vi "chipKIT UART2 Write.vi"() -> ()   [LabVIEW 2011, in "LabVIEW Interface for ChipKit.lvlib"]
doc: "Write serial data using the secondary UART on the chipKIT."
uses:
  vi.lib/LabVIEW Interface for ChipKit/LabVIEW Interface for ChipKit.lvlib
  vi.lib/LabVIEW Interface for ChipKit/Private/Type Defs/Chipkit Configuration.ctl
  vi.lib/LabVIEW Interface for ChipKit/Private/Type Defs/Board Type.ctl
panel:
  in  "Send":bool
  in  "Serial Data":string
  in  "Stop Button":bool
  in  "Buad Rate":u32=9600
  in  "ChipKit Configuration":T1={"COM Port"="COM3", "Board Type"=enum."ChipKit uC32"}
  # "UART2 Write Example\n\nThis example demonstrates how write serial data usring the secondary UART\non the chipKIT\n\nInstructions\n1. Select the COM Port associated with the ChipKit.\n2. Select the Board Type.\n3. Select the Baud Rate for thes secondary UART.\n4. Click the Run Arrow.\n5. Enter a value into the Serial Data string control.\n6. Click Send."
  # "chipKIT Settings"
  # "Channel Settings"
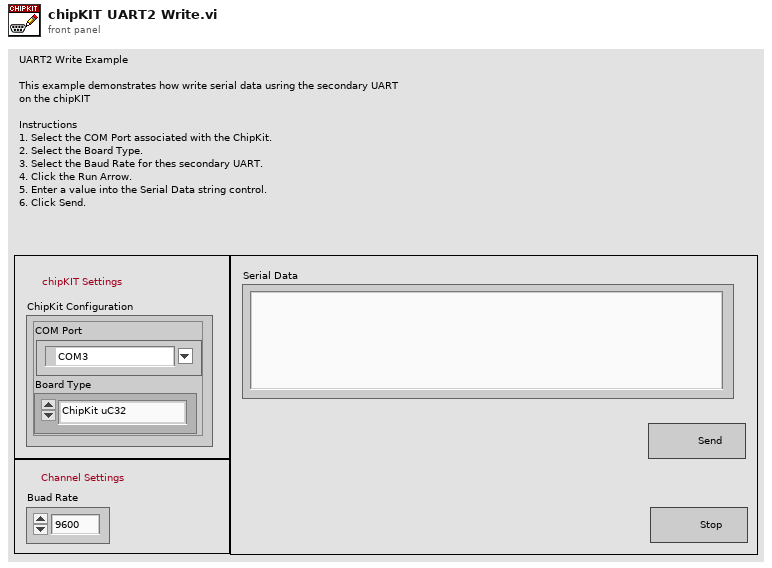
[diagram p1: front panel]
types:
  T1 = typedef "LabVIEW Interface for ChipKit.lvlib/Chipkit Configuration.ctl" = cluster{"COM Port":refnum<visa-resource-name>, "Board Type":T2}
  T2 = typedef "LabVIEW Interface for ChipKit.lvlib/Board Type.ctl" = enum16{"ChipKit uC32", "ChipKit Uno32", "ChipKit Max32"}
  T3 = typedef "LabVIEW Interface for ChipKit.lvlib/Chipkit Resource.ctl" = cluster{"COM Port":refnum<visa-resource-name>, "Board Type":T2, "Connection Type":T4, "Baud Rate (115200)":u32, "Bytes Per Packet (15)":u32, "DI Port Num Pins":i32, "DO Port Num Pins":i32}
  T4 = typedef "LabVIEW Interface for ChipKit.lvlib/Connection Type.ctl" = enum8{"USB / Serial", "XBEE", "BlueSmirf (Bluetooth)"}
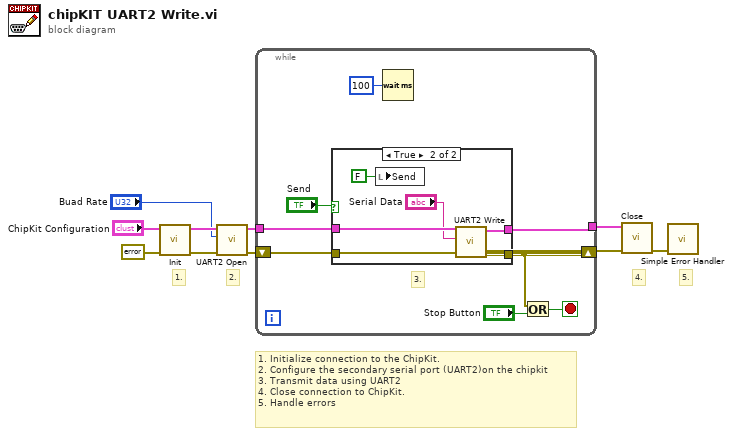
[diagram p0: block diagram]
diagram:
  # "1. Initialize connection to the ChipKit.\n2. Configure the secondary serial port (UART2)on the chipkit\n3. Transmit data using UART2\n4. Close connection to ChipKit.\n5. Handle errors"
  # "5."
  # "4."
  # "2."
  # "1."
  n1 = call "Init.vi"("Error In"=errorcluster {"status"=FALSE, "code"=0, "source"=""}, "ChipKit Configuration"="ChipKit Configuration") -> ("Error Out"=w6:errorcluster, "ChipKit Configuration"=w10:T3)  [unwired: 8 in]
  n2 = call "UART2 Open.vi"("Error In"=w6, "Buad Rate"="Buad Rate", "ChipKit Resource"=w10) -> ("Error Out"=w7:errorcluster, "ChipKit Resource"=w9:T3)  [unwired: 7 in]
  n3 = while {
    tunnel: w9 -> [w15]
    shift-right: [w11] -> w8
    shift-left: w7 -> [w14]
    tunnel: [w12] -> w1
    stop <- w17 stop-if-true
    # "3."
    n4 = case shown="True" "Send" {
      tunnel: w15 -> [w20 w26]
      tunnel: w14 -> [w19 w25]
      tunnel: [w20 w22] -> w12
      tunnel: [w19 w21] -> w11
      frame False {
      }
      frame True {
        n5 = local write "Send"(FALSE ("Send")) -> ()
        n6 = call "UART2 Write.vi"("Error In"=w25, "Data"="Serial Data", "ChipKit Resource 2"=w26) -> ("Error Out"=w21:errorcluster, "ChipKit Resource"=w22:T3)  [unwired: 7 in]
      }
    }
    n7 = Wait (ms)(milliseconds to wait=u32 100) -> ()  [unwired: 1 out]
    n8 = Or(x=w11, y="Stop Button") -> (x .or. y?=w17:bool)
  }
  n9 = call "Close.vi"("Error In"=w8, "ChipKit Configuration"=w1) -> ("Error Out"=w2:errorcluster)  [unwired: 9 in]
  n10 = call <vilib>:"Simple Error Handler.vi"("error in (no error)"=w2) -> ()  [unwired: 4 in, 5 out]
